vi "CreateTempFolder.vi"(8 "error in (no error)":errorcluster, 10 "Project":string, 11 "Root In":path) -> (0 "error out":errorcluster, 3 "Root Out":path)   [LabVIEW 2019]
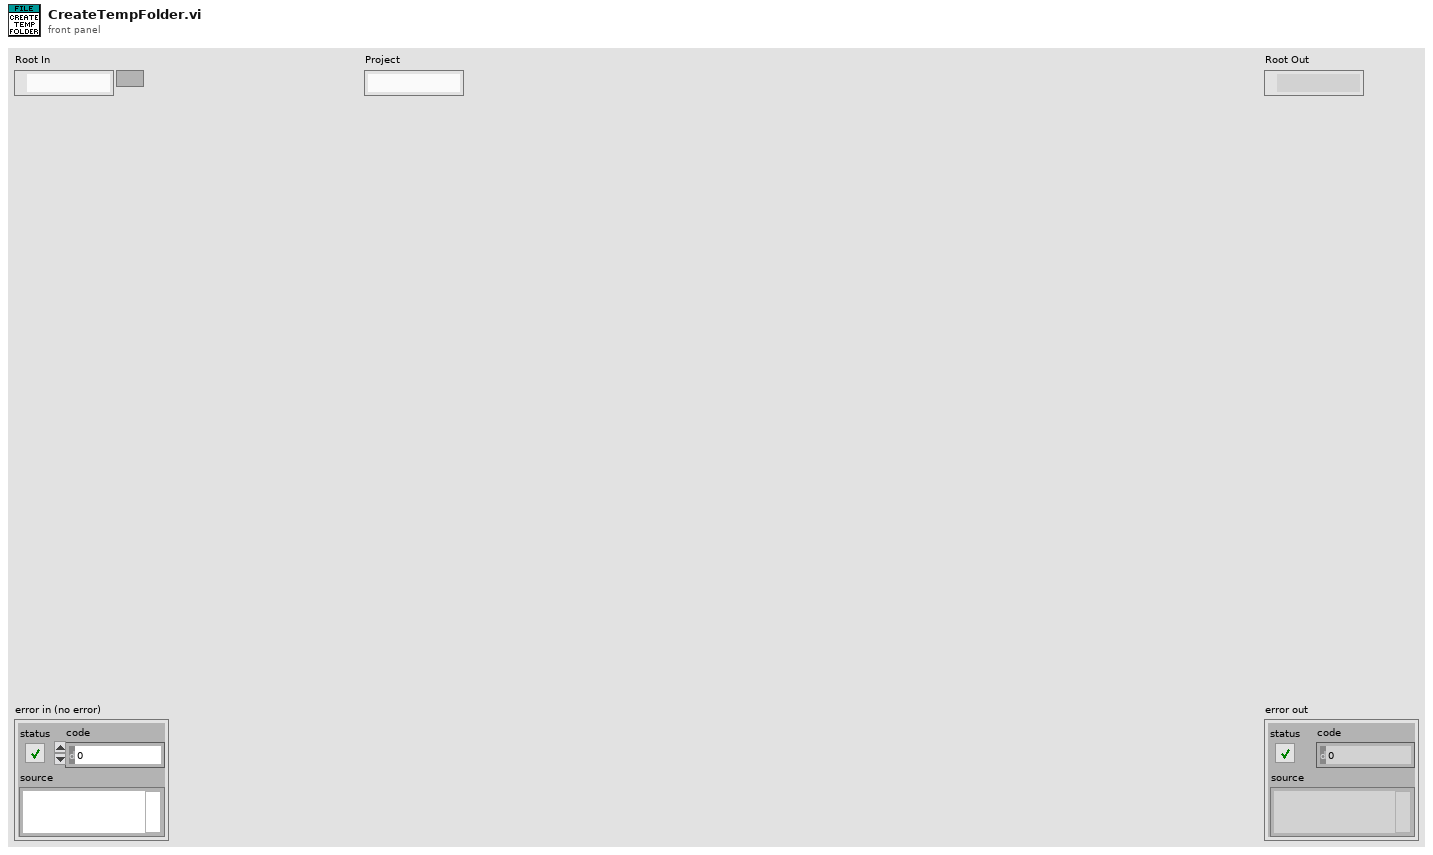
[diagram p1: front panel]
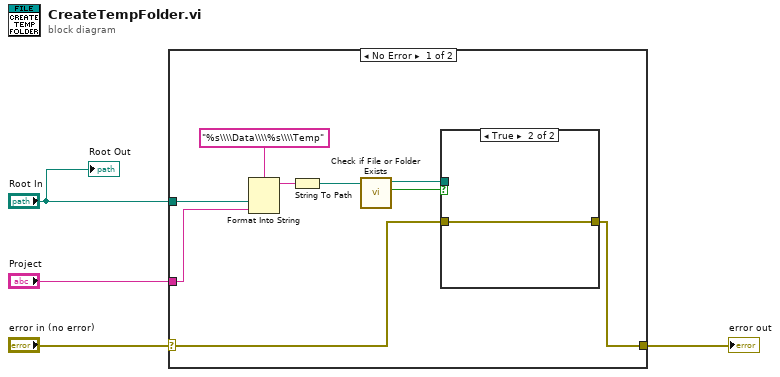
[diagram p0: block diagram]
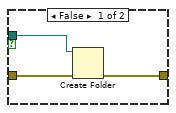
[diagram p2: hidden frame]
diagram:
  n1 = case shown="No Error" "error in (no error)" {
    selector: "error in (no error)" -> [w9 w18]
    tunnel: "Root In" -> [w13 _]
    tunnel: [w8 w18] -> w2
    tunnel: "Project" -> [w11 _]
    frame No Error {
      n2 = Format Into String(format string="%s\\\\Data\\\\%s\\\\Temp", w13, w11) -> (resulting string=w10:string)  [unwired: 2 in, 1 out]
      n3 = String To Path(string=w10) -> (path=w7:path)
      n4 = call <vilib>:"Check if File or Folder Exists.vi"("path"=w7) -> ("file or folder exists?"=w6:bool, "dup path"=w5:path)  [unwired: 8 in, 1 out]
      n5 = case shown="True" w6 {
        tunnel: w9 -> [w16 w17]
        tunnel: [w15 w17] -> w8
        tunnel: w5 -> [w14 _]
        frame False {
          n6 = Create Folder(path (use dialog)=w14, error in=w16) -> (error out=w15:errorcluster)  [unwired: 1 in, 2 out]
        }
        frame True {
        }
      }
    }
    frame Error {
    }
  }
  "error out" <- w2
  "Root Out" <- "Root In"
